vi "十进制转换为33进制-联想.vi"(11 "input_SN":string) -> (3 "show_str":string)   [LabVIEW 2011]
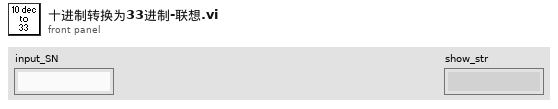
[diagram p1: front panel]
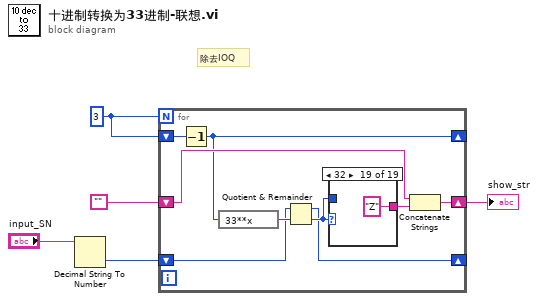
[diagram p0: block diagram]
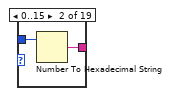
[diagram p3: hidden frame]
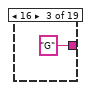
[diagram p4: hidden frame]
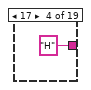
[diagram p5: hidden frame]
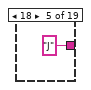
[diagram p6: hidden frame]
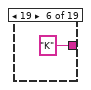
[diagram p7: hidden frame]
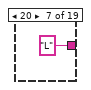
[diagram p8: hidden frame]
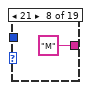
[diagram p9: hidden frame]
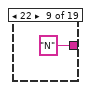
[diagram p10: hidden frame]
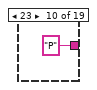
[diagram p11: hidden frame]
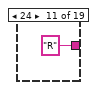
[diagram p12: hidden frame]
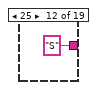
[diagram p13: hidden frame]
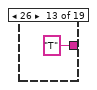
[diagram p14: hidden frame]
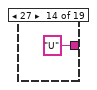
[diagram p15: hidden frame]
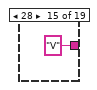
[diagram p16: hidden frame]
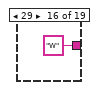
[diagram p17: hidden frame]
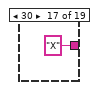
[diagram p18: hidden frame]
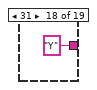
[diagram p19: hidden frame]
diagram:
  w4 = 3
  # "除去IOQ"
  n1 = Decimal String To Number(string="input_SN") -> (number=w5:i32)  [unwired: 2 in, 1 out]
  n2 = for {
    N: w4 -> [_]
    shift-right: [w10] -> w1
    shift-left: "" -> [w11]
    shift-right: [w8] -> _
    shift-left: w4 -> [w9]
    shift-right: [w6] -> _
    shift-left: w5 -> [w7]
    n3 = Decrement(x=w9) -> (x-1=w8:i32)
    n4 = expression code="33**x"(w8) -> (w14:i32)
    n5 = Quotient & Remainder(x=w7, y=w14) -> (x-y*floor(x/y)=w6:i32, floor(x/y)=w13:i32)
    n6 = case shown="32" w13 {
      tunnel: w13 -> [_ w16 _ _ _ _ _ _ _ _ _ _ _ _ _ _ _ _ _]
      tunnel: [_ w15 "G" "H" "J" "K" "L" "M" "N" "P" "R" "S" "T" "U" "V" "W" "X" "Y" "Z"] -> w12
      frame Default {
      }
      frame 0..15 {
        n7 = Number To Hexadecimal String(2:w16) -> (0:w15:string)  [unwired: 1 in]
      }
      frame 16 {
      }
      frame 17 {
      }
      frame 18 {
      }
      frame 19 {
      }
      frame 20 {
      }
      frame 21 {
      }
      frame 22 {
      }
      frame 23 {
      }
      frame 24 {
      }
      frame 25 {
      }
      frame 26 {
      }
      frame 27 {
      }
      frame 28 {
      }
      frame 29 {
      }
      frame 30 {
      }
      frame 31 {
      }
      frame 32 {
      }
    }
    n8 = Concatenate Strings(w11, w12) -> (w10:string)
  }
  "show_str" <- w1
